vi "ReadFileVersion.vi"(8 "error in (no error)":errorcluster, 11 "object in":refnum<class "SequenceManager.lvclass">) -> (0 "error out":errorcluster, 2 "FileVersion":string, 3 "object out":refnum<class "SequenceManager.lvclass">)   [LabVIEW 2023, in "Easy.SequenceManagerLabVIEW.lvlib" / "SequenceManager.lvclass"]
uses:
  SequenceManager.lvclass
  SequenceManager.lvclass/SequenceManager.ctl
panel:
  # "Connector Pane"
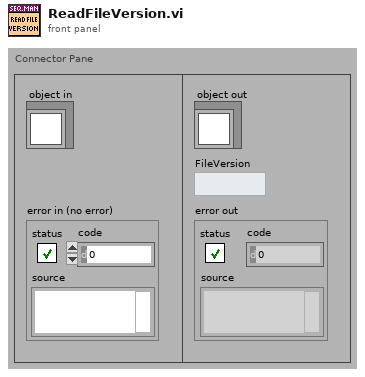
[diagram p1: front panel]
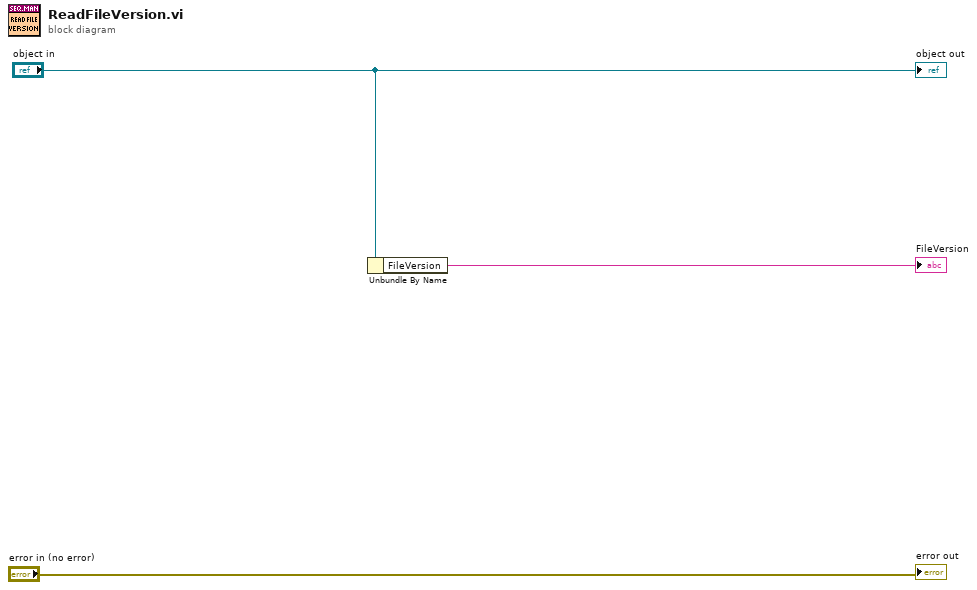
[diagram p0: block diagram]
diagram:
  n1 = Unbundle By Name("object in") -> ("FileVersion"=→"FileVersion":string)
  "error out" <- "error in (no error)"
  "object out" <- "object in"
